vi "Application.vi"(1 "Trial Length (S)":dbl=5.0 min=0.0 step=1.0, 12 "stop (T)":bool=TRUE caption="stop") -> ()   [LabVIEW 2017]
uses:
  <vilib>/addons/_NISVFA/_Shared subVIs/Controls/svc_Window [Dual FFT].ctl
  <vilib>/DAQmx/read.llb/DAQmx Read (Analog 1D DBL NChan 1Samp).vi
  <vilib>/DAQmx/configure/timing.llb/DAQmx Timing (Sample Clock).vi
  <vilib>/DAQmx/create/channels.llb/DAQmx Create Channel (AI-Voltage-Basic).vi
panel:
  in  "Tab Control 5":enum32{"Acquisition", "Results"}(tab)
  out "elapsed time":dbl format="%.2f"
  in  "Lead In":tag="Dev2/ai0"
  in  "Lead Out":tag="Dev2/ai1"
  in  "Trail Out":tag="Dev2/ai3"
  in  "Trail In":tag="Dev2/ai2"
  in  "simulation":bool=TRUE caption="sample clock"
  out "file preview":string
  out "Progress %":dbl(slide) scale=0.0..100.0
  in  "Acquisition Source":enum32{"Device Acquistion", "File Input"}(radio)
  out "Write Path":path
  out "timestamp":string
  in  "file name":string
  out "ai0 Chart":dbl(graph)
  out "ai1 Chart":dbl(graph)
  out "ai2 Chart":dbl(graph)
  out "ai3 Chart":dbl(graph)
  in  "Tab Control":T1(tab)
  out "Raw Signal TA":waveform(dbl)(graph) caption="Waveform Graph"
  out "FFT TA":cluster{"X":dbl, "Y":dbl}[](graph)
  out "dB On 6":bool=TRUE
  out "unit label 9":string
  out "frequency range 8":T2={"low band"=enum."20 Hz", "high band"=enum."20000 Hz"}
  out "octave graph":T3(graph)
  out "total band power [dB] 4":dbl=nan format="%.9f"
  out "RMS [V^2]\nBands [Hz] 5":dbl[][](array[numeric])
  out "unit label":string
  out "frequency range 9":T2={"low band"=enum."20 Hz", "high band"=enum."20000 Hz"}
  out "dB On  2":bool=TRUE
  out "octave graph 2":T3(graph)
  out "total band power [dB EU]":dbl=nan format="%.2f"
  out "SPL [dB]\nBands [Hz]":dbl[][](array[numeric])
  out "SPL [dB] TA":dbl
  out "RMS FFT TA":dbl
  out "Trailing Edge Probe – Mic A":string
  out "Trailing Edge Probe – Mic B":string
  out "Leading Edge Probe – Mic A":string
  out "Leading Edge Probe – Mic B":string
  in  "Tab Control 3":T4(tab) caption="Tab Control"
  out "Raw Signal LA 2":waveform(dbl)(graph) caption="Waveform Graph"
  out "FFT LA":cluster{"X":dbl, "Y":dbl}[](graph)
  out "unit label":string
  out "frequency range RMS 3":T2={"low band"=enum."20 Hz", "high band"=enum."20000 Hz"}
  out "dB On":bool=TRUE
  out "octave graph":T3(graph)
  out "RMS [V^2]\nBands [Hz]":dbl[][](array[numeric])
  out "total band power [dB]":dbl=nan format="%.7f"
  out "unit label":string
  out "dB On 7":bool=TRUE
  out "frequency range":T2={"low band"=enum."20 Hz", "high band"=enum."20000 Hz"}
  out "octave graph 5":T3(graph)
  out "SPL [dB]\nBands [Hz]":dbl[][](array[numeric])
  out "total band power [dB EU]":dbl=nan format="%.2f"
  out "SPL [dB] LA 2":dbl
  out "RMS FFT LA":dbl
  in  "Tab Control 4":T4(tab) caption="Tab Control"
  out "Raw Signal LB":waveform(dbl)(graph) caption="Waveform Graph"
  out "FFT LB":cluster{"X":dbl, "Y":dbl}[](graph)
  out "unit label 10":string
  out "dB On 2":bool=TRUE
  out "frequency range":T2={"low band"=enum."20 Hz", "high band"=enum."20000 Hz"}
  out "octave graph 8":T3(graph)
  out "RMS [V^2]\nBands [Hz]":dbl[][](array[numeric])
  out "total band power [V^2]":dbl=nan format="%.7f"
  out "dB On":bool=TRUE
  out "frequency range":T2={"low band"=enum."20 Hz", "high band"=enum."20000 Hz"}
  out "unit label 11":string
  out "octave graph 7":T3(graph)
  out "SPL [dB]\nBands [Hz] 2":dbl[][](array[numeric])
  out "total band power [dB]":dbl=nan format="%.2f"
  out "SPL [dB] LB":dbl
  out "RMS FFT LB":dbl
  in  "Select Probe:":string(combo)
  out "DATA":string
  out "Single Probe SPL Log Avg:":dbl[][](array[numeric])
  out "Single Probe Coherence [dB EU]":dbl[](array[numeric]) format="%_9g"
  out "Entire-Spectrum Single-Probe SPL [dB]":dbl
  out "Overall SPL Log Avg:":dbl[][](array[numeric])
  out "Entire-Spectrum Overall SPL [dB]:":dbl
  in  "Tab Control 2":T4(tab) caption="Tab Control"
  out "Raw Signal TB":waveform(dbl)(graph) caption="Waveform Graph"
  out "FFT TB":cluster{"X":dbl, "Y":dbl}[](graph)
  out "unit label":string
  out "dB On 5":bool=TRUE
  out "frequency range":T2={"low band"=enum."20 Hz", "high band"=enum."20000 Hz"}
  out "octave graph":T3(graph)
  out "total band power [dB EU]":dbl=nan format="%.7f"
  out "RMS [V^2]\nBands [Hz]":dbl[][](array[numeric])
  out "unit label":string
  out "dB On":bool=TRUE
  out "frequency range":T2={"low band"=enum."20 Hz", "high band"=enum."20000 Hz"}
  out "octave graph":T3(graph)
  out "SPL [dB]\nBands [Hz]":dbl[][](array[numeric])
  out "total band power [dB EU]":dbl=nan format="%.2f"
  out "SPL [dB] TB":dbl
  out "RMS FFT TB":dbl
  out "octave spectrum 4":T5 {"band power" format="%.2f"; "nominal frequencies [Hz]" format="%.2f"}
  # "SPL [dB]"
  # "Band [Hz]"
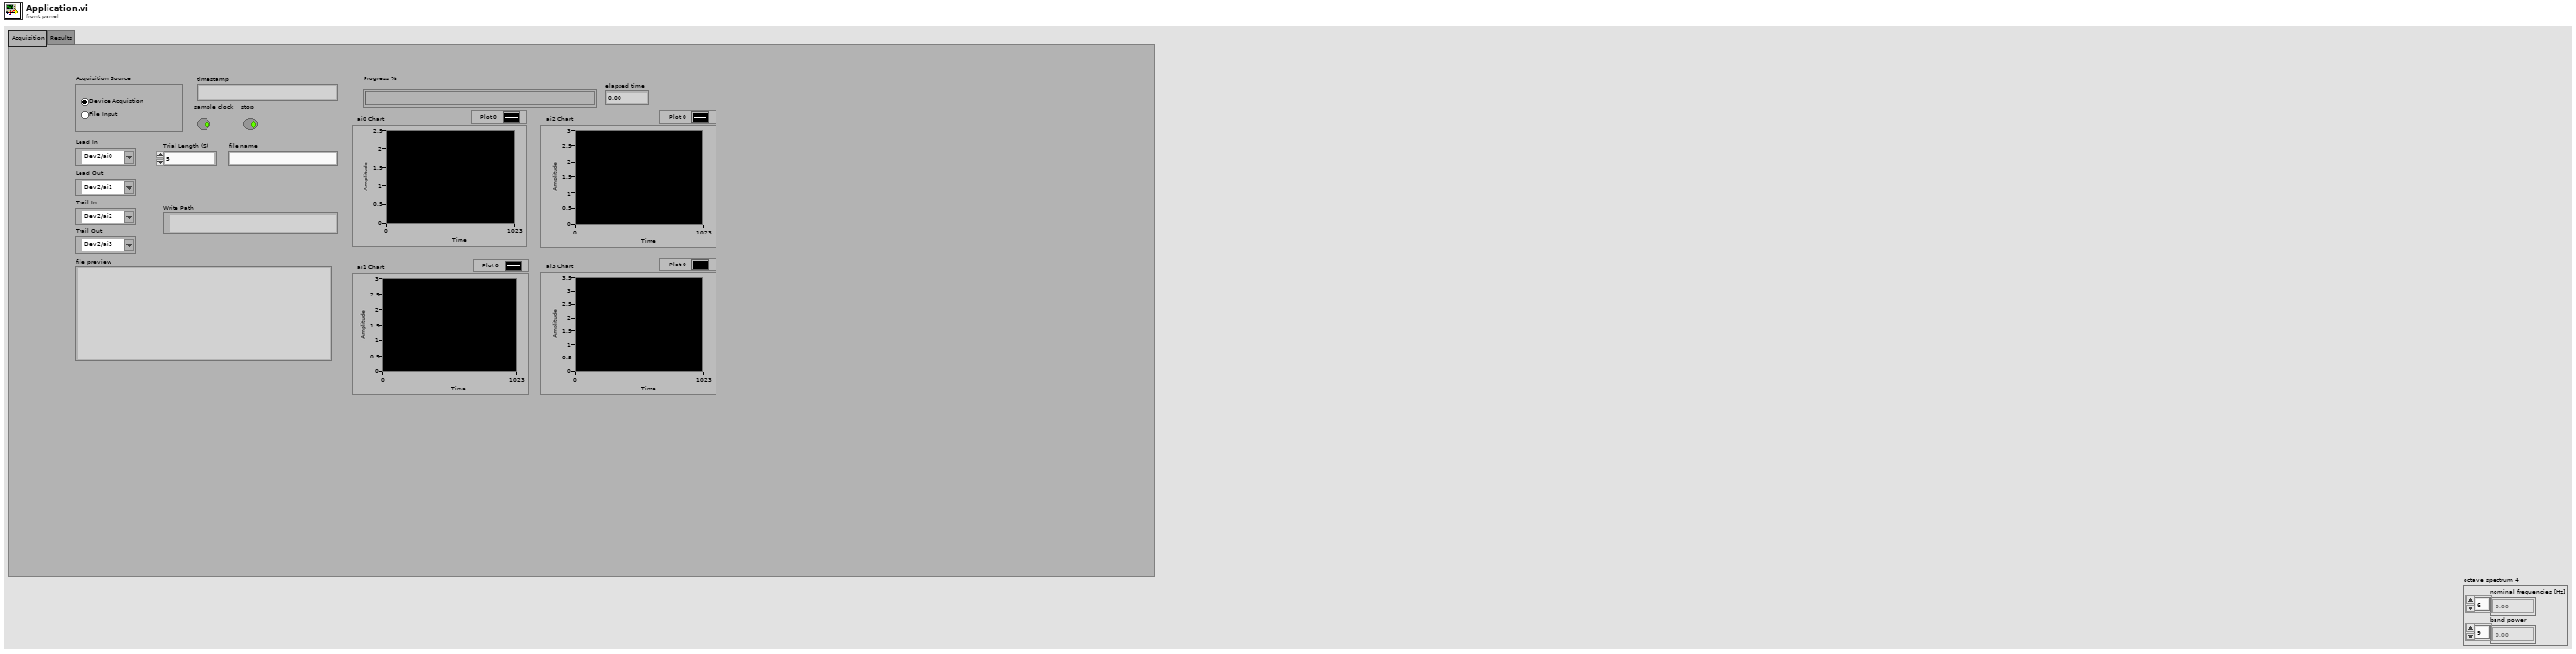
[diagram p1: front panel]
types:
  T1 = enum32{"Raw Signal", "FFT", "FFT Phase", "RMS Graph", "RMS Data", "SPL Graph", "SPL Data", "Full Spectrum Data"}
  T2 = cluster{"low band":enum16{"20 Hz", "25 Hz", "31.5 Hz", "40 Hz", "50 Hz", "63 Hz", "80 Hz", "100 Hz", "125 Hz", "160 Hz", "200 Hz", "250 Hz", "315 Hz", "400 Hz", "500 Hz", "630 Hz", "800 Hz", "1000 Hz", "1250 Hz", "1600 Hz", "2000 Hz", "2500 Hz", "3150 Hz", "4000 Hz", "5000 Hz", "6300 Hz", "8000 Hz", "10000 Hz", "12500 Hz", "16000 Hz", "20000 Hz"}, "high band":enum16{"20 Hz", "25 Hz", "31.5 Hz", "40 Hz", "50 Hz", "63 Hz", "80 Hz", "100 Hz", "125 Hz", "160 Hz", "200 Hz", "250 Hz", "315 Hz", "400 Hz", "500 Hz", "630 Hz", "800 Hz", "1000 Hz", "1250 Hz", "1600 Hz", "2000 Hz", "2500 Hz", "3150 Hz", "4000 Hz", "5000 Hz", "6300 Hz", "8000 Hz", "10000 Hz", "12500 Hz", "16000 Hz", "20000 Hz"}}
  T3 = cluster{"nominal frequencies [Hz]":dbl[], "band power [dB EU]":dbl[]}
  T4 = enum32{"Raw Signal", "FFT", "RMS Graph", "RMS Data", "SPL Graph", "SPL Data", "Full Spectrum Data"}
  T5 = cluster{"nominal frequencies [Hz]":dbl[], "band power":dbl[]}
  T6 = enum16{"Linear", "Exponential", "Equal confidence", "Peak"}
  T7 = typedef "svc_Window [Dual FFT].ctl" = u32
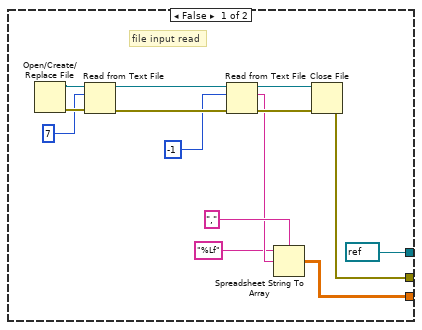
[diagram p2: hidden frame]
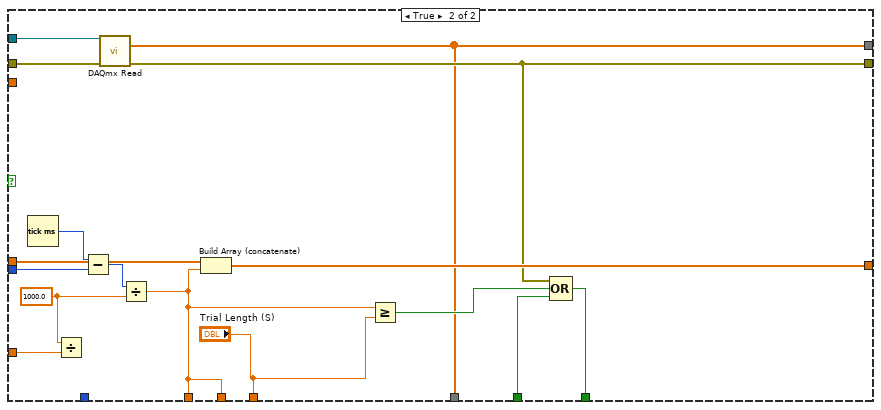
[diagram p4: hidden frame]
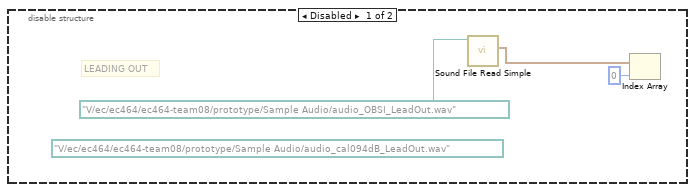
[diagram p6: hidden frame]
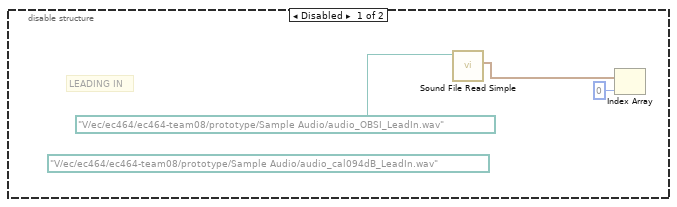
[diagram p7: hidden frame]
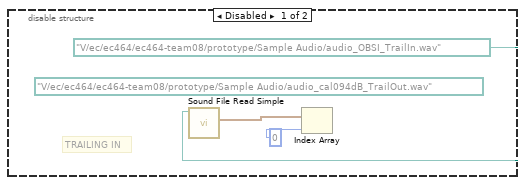
[diagram p9: hidden frame]
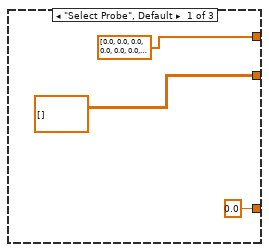
[diagram p10: hidden frame]
diagram:
  n1 = flat-sequence {
    tunnel: [w31] -> w2
    tunnel: [w30] -> w1
    tunnel: [w56] -> w12
    tunnel: [w55] -> w10
    tunnel: [w54] -> w8
    tunnel: [w53] -> w6
    tunnel: [w52] -> w4
    tunnel: w2 -> [w51]
    tunnel: w1 -> [w50]
    tunnel: [w98] -> w14
    tunnel: [w97] -> w13
    tunnel: w12 -> [w97]
    tunnel: [w96] -> w11
    tunnel: w10 -> [w96]
    tunnel: [w95] -> w9
    tunnel: w8 -> [w95]
    tunnel: [w94] -> w7
    tunnel: w6 -> [w94]
    tunnel: [w93] -> w5
    tunnel: w4 -> [w93]
    tunnel: [w92] -> w3
    tunnel: [w118] -> w29
    tunnel: [w117] -> w28
    tunnel: [w113] -> w27
    tunnel: [w116] -> w23
    tunnel: [w115] -> w22
    tunnel: [w114] -> w18
    tunnel: [w111] -> w15
    tunnel: w14 -> [w111]
    tunnel: w13 -> [w110]
    tunnel: w11 -> [w109]
    tunnel: w9 -> [w108]
    tunnel: w7 -> [w107]
    tunnel: w5 -> [w106]
    tunnel: w3 -> [w105]
    tunnel: w29 -> [w188]
    tunnel: [w188] -> w24
    tunnel: [w187] -> w25
    tunnel: w28 -> [w187]
    tunnel: w27 -> [w186]
    tunnel: [w186] -> w26
    tunnel: w23 -> [w185]
    tunnel: w22 -> [w181]
    tunnel: w18 -> [w184]
    tunnel: [w184] -> w17
    tunnel: [w183] -> w16
    tunnel: w15 -> [w183]
    tunnel: [w332] -> w21
    tunnel: [w331] -> w20
    tunnel: [w330] -> w19
    tunnel: w16 -> [w214]
    tunnel: w17 -> [_]
    tunnel: w24 -> [w330]
    tunnel: w25 -> [w331]
    tunnel: w26 -> [w332]
    tunnel: w21 -> [w358]
    tunnel: w20 -> [w359]
    tunnel: w19 -> [w356]
    frame #0 {
      w43 = 0 ("index")
      n2 = call <vilib>:"DAQmx Unflatten Channel String.vi"("names in"="Trail Out") -> ("names out"=w44:string[])  [unwired: 13 in, 1 out]
      n3 = call <vilib>:"DAQmx Unflatten Channel String.vi"("names in"="Trail In") -> ("names out"=w45:string[])  [unwired: 13 in, 1 out]
      n4 = call <vilib>:"DAQmx Unflatten Channel String.vi"("names in"="Lead In") -> ("names out"=w47:string[])  [unwired: 13 in, 1 out]
      n5 = call <vilib>:"DAQmx Unflatten Channel String.vi"("names in"="Lead Out") -> ("names out"=w46:string[])  [unwired: 13 in, 1 out]
      n6 = Index Array(array=w46, index=w43) -> (element=w41:string)
      n7 = Index Array(array=w45, index=w43) -> (element=w40:string)
      n8 = Index Array(array=w47, index=w43) -> (element=w42:string)
      n9 = Index Array(array=w44, index=w43) -> (element=w39:string)
      n10 = call "append channels"("Trail Out"=w39, "Lead In"=w42, "Lead Out"=w41, "Trail In"=w40) -> ("Result"=w31:string, "error out"=w30:errorcluster)  [unwired: 10 in]
      "Trailing Edge Probe – Mic A" <- "Trailing Edge Probe – Mic A"
      "Trailing Edge Probe – Mic B" <- "Trailing Edge Probe – Mic B"
      "Leading Edge Probe – Mic A" <- "Leading Edge Probe – Mic A"
      "Leading Edge Probe – Mic B" <- "Leading Edge Probe – Mic B"
      "DATA" <- "DATA" ("DATA")
    }
    frame #1 {
      w52 = 16384.0 ("y")
      n11 = Equal To 0?(x="Acquisition Source") -> (x = 0?=w56:bool)
      n12 = case shown="True" w56 {
        tunnel: [refnum<k21> refnum ("task out") w81] -> w55
        tunnel: [w62 w80] -> w54
        tunnel: w52 -> [_ w76]
        tunnel: [w58 dbl[][] []] -> w53
        tunnel: w51 -> [_ w72]
        tunnel: w50 -> [_ w73]
        frame False {
          # "file input read"
          n13 = Open/Create/Replace File() -> (refnum out=w70:refnum<file>, error out=w69:errorcluster)  [unwired: 6 in, 1 out]
          n14 = Read from Text File(file (use dialog)=w70, count=7, error in=w69) -> (refnum out=w67:refnum<file>, error out=w64:errorcluster)  [unwired: 1 in, 2 out]
          n15 = Read from Text File(file (use dialog)=w67, count=-1, error in=w64) -> (refnum out=w66:refnum<file>, text=w60:string, error out=w65:errorcluster)  [unwired: 1 in, 1 out]
          n16 = Spreadsheet String To Array(delimiter (Tab)=",", format string="%Lf", spreadsheet string=w60) -> (array=w58:dbl[][])  [unwired: 1 in]
          n17 = Close File(refnum=w66, error in=w65) -> (error out=w62:errorcluster)  [unwired: 1 out]
        }
        frame True {
          w79 = 10348 items=["Volts"=10348, "From Custom Scale"=10065] ("units")
          n18 = call-poly <vilib>:"DAQmx Create Virtual Channel.vi"("physical channels"=w72, "units"=w79, "error in"=w73) -> ("task out"=w78:refnum<k21>, "error out"=w77:errorcluster)  [unwired: 11 in]
          n19 = case shown="True" "simulation" {
            tunnel: [w83 w91] -> w81
            tunnel: [w82 w90] -> w80
            tunnel: w78 -> [w83 w89]
            tunnel: w77 -> [w82 w88]
            tunnel: w76 -> [_ w85]
            frame False {
            }
            frame True {
              w87 = 10178 items=["Finite Samples"=10178, "Continuous Samples"=10123, "Hardware Timed Single Point"=12522] ("sample mode")
              n20 = local read "Trial Length (S)"() -> (w86:dbl)
              n21 = Multiply(x=w86, y=w85) -> (x*y=w84:dbl)
              n22 = call-poly <vilib>:"DAQmx Timing.vi"("task/channels in"=w89, "sample mode"=w87, "samples per channel"=w84, "rate"=w85, "error in"=w88) -> ("task out"=w91:refnum<k21>, "error out"=w90:errorcluster)  [unwired: 9 in]
            }
          }
        }
      }
    }
    frame #2 {
      # "Get the timestamp"
      n23 = Get Date/Time In Seconds() -> (seconds since 1Jan1904=w98:timestamp)
      n24 = Tick Count (ms)() -> (millisecond timer value=w92:u32)
      n25 = Get Date/Time String(date format (0)=enum16{"short", "long", "abbreviated"}."long", seconds (now)=w98, want seconds? (F)=TRUE) -> (date string=w102:string, time string=w104:string)
      n26 = call <vilib>:"Space Constant.vi"() -> ("String"=w103:string)
      n27 = Concatenate Strings(w102, w103, w104) -> (→"timestamp":string)
    }
    frame #3 {
      n28 = while {
        shift-right: [w143] -> w117
        shift-left: dbl[] [] -> [w146]
        tunnel: [w137] -> w118 mode=indexing
        tunnel: [w137] -> w114
        tunnel: [w142] -> w115
        tunnel: [w130] -> w113 mode=indexing
        tunnel: w110 -> [w124]
        tunnel: w109 -> [w123]
        tunnel: w108 -> [w122]
        tunnel: w107 -> [w121]
        tunnel: w106 -> [w120]
        tunnel: w105 -> [w119]
        i -> [w137]
        stop <- w144 stop-if-true
        # "TO"
        # "TI"
        # "LO"
        # "LI"
        n29 = case shown="False" w124 {
          tunnel: w146 -> [_ w179]
          tunnel: w119 -> [w153 w169]
          tunnel: "stop (T)" -> [w163 w178]
          tunnel: [w162 w177] -> w144
          tunnel: [w152 w176] -> w143
          tunnel: w123 -> [_ w175]
          tunnel: w122 -> [w164 w174]
          tunnel: [w151 w171] -> w130
          tunnel: [w164 w173] -> w142
          tunnel: w120 -> [_ w172]
          tunnel: [w155 w165] -> w136
          tunnel: [w154 "Trial Length (S)"] -> w140
          tunnel: w121 -> [w160 _]
          tunnel: w137 -> [w155 _]
          tunnel: [w147 w165] -> w135
          tunnel: [w151 w171] -> w129
          frame False {
            # "file input parse"
            n30 = Tick Count (ms)() -> (millisecond timer value=w150:u32)
            n31 = Subtract(x=w150, y=w153) -> (x-y=w149:u32)
            n32 = Divide(x=w149, y=1000.0 ("x")) -> (x/y=w147:dbl)
            n33 = Index Array(array=w160, index (row)=w155) -> (element=w157:dbl[])  [unwired: 1 in]
            n34 = Index Array(array=w160, index (col)=1 ("disabled index (col)")) -> (element=w152:dbl[])  [unwired: 1 in]
            n35 = Array Subset(array=w157, index=2, length=4) -> (w151:dbl[])
            n36 = Array Size(array=w152) -> (size(s)=w154:i32)
            n37 = Greater Or Equal?(x=w155, y=w154) -> (x >= y?=w156:bool)
            n38 = Compound Arithmetic op=OR(w156, w163) -> (w162:bool)
          }
          frame True {
            w167 = 1000.0 ("x")
            n39 = Tick Count (ms)() -> (millisecond timer value=w168:u32)
            n40 = Divide(x=w167, y=w172) -> ()  [unwired: 1 out]
            n41 = Subtract(x=w168, y=w169) -> (x-y=w166:u32)
            n42 = call-poly <vilib>:"DAQmx Read.vi"("task/channels in"=w175, "error in"=w174) -> ("data"=w171:dbl[], "error out"=w173:errorcluster)  [unwired: 11 in, 1 out]
            n43 = Divide(x=w166, y=w167) -> (x/y=w165:dbl)
            n44 = Build Array (concatenate)(w179, w165) -> (w176:dbl[])
            n45 = Greater Or Equal?(x=w165, y="Trial Length (S)") -> (x >= y?=w180:bool)
            n46 = Compound Arithmetic op=OR(w173, w180, w178) -> (w177:bool)
          }
        }
        "elapsed time" <- w135
        n47 = Divide(x=w136, y=w140) -> (x/y=w139:dbl)
        n48 = Multiply(x=w139, y=100.0) -> (x*y=→"Progress %":dbl)
        n49 = Index Array(array=w129, index=2 ("disabled index (col)")) -> (element=→"ai2 Chart":dbl)
        n50 = Index Array(array=w129, index=3 ("disabled index (col)")) -> (element=→"ai3 Chart":dbl)
        n51 = Index Array(array=w129, index=0 ("disabled index (col)")) -> (element=→"ai0 Chart":dbl)
        n52 = Index Array(array=w129, index=1 ("disabled index (col)")) -> (element=→"ai1 Chart":dbl)
      }
      n53 = Equal To 0?(x=w114) -> (x = 0?=w116:bool)
    }
    frame #4 {
      n54 = Compound Arithmetic op=OR(w181, w185) -> (w182:bool)
      n55 = case shown="True" w182 {
        selector: w182 -> [w194 _]
        tunnel: w181 -> [w193 _]
        frame True {
          n56 = And(x=w194, y=w193) -> (x .and. y?=w196:bool)
          n57 = flat-sequence {
            tunnel: [w200] -> w197
            tunnel: w193 -> [w199]
            tunnel: w189 -> [w198]
            tunnel: w197 -> [w202]
            frame #0 {
              n58 = call "Display Message to User2"("error in (no error)"=w199, "Message"=w198) -> ("stop program"=w200:bool)  [unwired: 8 in, 1 out]
            }
            frame #1 {
              n59 = Or(x=TRUE, y=w202) -> (x .or. y?=w203:bool)
              n60 = Stop(stop? (T)=w203) -> ()
            }
          }
          n61 = call <vilib>:"Simple Error Handler.vi"() -> ("message"=w191:string)  [unwired: 5 in, 4 out]
          n62 = Select(t=w191, s=w196, f="Application Stopped, No Error.") -> (s? t:f=w190:string)
          n63 = Concatenate Strings("Application Error: ", w190) -> (w189:string)
        }
        frame False {
        }
      }
    }
    frame #5 {
      w205 = T7 1 items=["None"=0, "Hanning"=1, "Hamming"=2, "Blackman-Harris"=3, "Exact Blackman"=4, "Blackman"=5, "Flat Top"=6, "4 Term B-Harris "=7, "7 Term B-Harris"=8, "Low Sidelobe"=9, "Force - Exponential"=10, "Force"=64, "Exponential"=65, "Blackman Nuttall"=11, "Triangle"=30, "Bartlett-Hanning"=31, "Bohman"=32, "Parzen"=33, "Welch"=34, "Kaiser"=60, "Dolph-Chebyshev"=61, "Gaussian"=62] ("window")
      w207 = T7 1 items=["None"=0, "Hanning"=1, "Hamming"=2, "Blackman-Harris"=3, "Exact Blackman"=4, "Blackman"=5, "Flat Top"=6, "4 Term B-Harris "=7, "7 Term B-Harris"=8, "Low Sidelobe"=9, "Force - Exponential"=10, "Force"=64, "Exponential"=65, "Blackman Nuttall"=11, "Triangle"=30, "Bartlett-Hanning"=31, "Bohman"=32, "Parzen"=33, "Welch"=34, "Kaiser"=60, "Dolph-Chebyshev"=61, "Gaussian"=62] ("window")
      # "dt"
      # "t0"
      # "SPL"
      # "RMS"
      # "LEADING"
      # "OVERALL SPL LOG AVG"
      # "ENTIRE SPECTRUM SINGLE PROBE SPL LOG SUM"
      # "TRAILING"
      # "RMS"
      # "SPL"
      # "ACROSS PROBE AVERAGED SPL"
      # "RMS"
      # "SPL"
      # "ACROSS PROBE AVERAGED SPL"
      # "RMS"
      # "SPL"
      # "TO"
      # "TI"
      # "LO"
      # "LI"
      n64 = Reciprocal(x=16384.0 ("y")) -> (1/x=w211:dbl)
      n65 = disable-structure shown="Enabled" {
        frame Disabled {
          (unwired) path "V:/ec/ec464/ec464-team08/prototype/Sample Audio/audio_cal094dB_TrailOut.wav" ("path")
          # "TRAILING IN"
          n66 = call <vilib>:"Sound File Read Simple.vi"("path"=path "V:/ec/ec464/ec464-team08/prototype/Sample Audio/audio_OBSI_TrailIn.wav") -> ("data"=w342:waveform(dbl)[])  [unwired: 7 in, 3 out]
          n67 = Index Array(array=w342, index=0) -> ()  [unwired: 1 out]
        }
        frame Enabled {
        }
      }
      n68 = Index Array(array=w332, index (col)=0 ("disabled index (col)")) -> (element=w213:dbl[])  [unwired: 1 in]
      n69 = Index Array(array=w332, index (col)=2 ("disabled index (col)")) -> (element=w212:dbl[])  [unwired: 1 in]
      n70 = Index Array(array=w332, index (col)=3 ("disabled index (col)")) -> (element=w209:dbl[])  [unwired: 1 in]
      n71 = Index Array(array=w332, index (col)=1 ("disabled index (col)")) -> (element=w218:dbl[])  [unwired: 1 in]
      n72 = Bundle By Name("t0"=w214, "dt"=w211, "Y"=w213) -> (w215:waveform(dbl))  [unwired: 1 in]
      "Raw Signal LA 2" <- w215
      n73 = Bundle By Name("t0"=w214, "dt"=w211, "Y"=w218) -> (w217:waveform(dbl))  [unwired: 1 in]
      "Raw Signal LB" <- w217
      n74 = Bundle By Name("t0"=w214, "dt"=w211, "Y"=w212) -> (w208:waveform(dbl))  [unwired: 1 in]
      "Raw Signal TA" <- w208
      n75 = Bundle By Name("t0"=w214, "dt"=w211, "Y"=w209) -> (w210:waveform(dbl))  [unwired: 1 in]
      "Raw Signal TB" <- w210
      n76 = call "EntireSpectrumProcess.vi"("data"=w208) -> ("RMS"=→"RMS FFT TA":dynamicdata, "Dynamic Data"=→"SPL [dB] TA":dynamicdata, "Array"=→"FFT TA":cluster{dbl, dbl}[])  [unwired: 8 in]
      n77 = call "OctaveBandsProcess.vi"("averaging type"=T6."Linear", "data"=w208, "dB On (T)"=FALSE) -> ("nominal frequencies [Hz]"=w309:dbl[], "frequency range"=→"frequency range 8":T2, "band power"=w289:dbl[], "octave spectrum"=→"octave graph":T5, "dB On"=→"dB On 6":bool, "unit label"=w287:string, "total band power"=→"total band power [dB] 4":dbl)  [unwired: 5 in, 1 out]
      "unit label 9" <- w287
      n78 = call "OctaveBandsProcess.vi"("averaging type"=T6."Linear", "data"=w208, "dB On (T)"=TRUE) -> ("nominal frequencies [Hz]"=w298:dbl[], "frequency range"=→"frequency range 9":T2, "band power"=w291:dbl[], "octave spectrum"=→"octave graph 2":T5, "dB On"=→"dB On  2":bool, "unit label"=w281:string, "total band power"=→"total band power [dB EU]":dbl)  [unwired: 5 in, 1 out]
      "unit label" <- w281
      n79 = property on="octave graph 2" class="XYGraph (strict)"("Y Scale.Name Label.Text"=w281) -> ()  [unwired: 2 in, 2 out]
      n80 = property on="octave graph" class="XYGraph (strict)"("Y Scale.Name Label.Text"=w287) -> ()  [unwired: 2 in, 2 out]
      n81 = disable-structure shown="Disabled" {
        frame Disabled {
          (unwired) path "V:/ec/ec464/ec464-team08/prototype/Sample Audio/audio_cal094dB_TrailOut.wav" ("path")
          # "TRAILING OUT"
          n82 = call <vilib>:"Sound File Read Simple.vi"("path"=path "V:/ec/ec464/ec464-team08/prototype/Sample Audio/audio_OBSI_TrailOut.wav") -> ("data"=w339:waveform(dbl)[])  [unwired: 7 in, 3 out]
          n83 = Index Array(array=w339, index=0) -> ()  [unwired: 1 out]
        }
        frame Enabled {
        }
      }
      n84 = Build Array(w291, w298) -> (→"SPL [dB]\nBands [Hz]":dbl[][])
      n85 = Build Array(w289, w309) -> (→"RMS [V^2]\nBands [Hz] 5":dbl[][])
      n86 = call "OctaveBandsProcess.vi"("averaging type"=T6."Linear", "data"=w210, "dB On (T)"=FALSE) -> ("nominal frequencies [Hz]"=w306:dbl[], "frequency range"=→"frequency range":T2, "band power"=w290:dbl[], "octave spectrum"=→"octave graph":T5, "dB On"=→"dB On 5":bool, "unit label"=w272:string, "total band power"=→"total band power [dB EU]":dbl)  [unwired: 5 in, 1 out]
      "unit label" <- w272
      n87 = call <vilib>:"SVFA Coherent Output Power.vi"("scaled signal X [EUx]"=w289, "scaled signal Y [EUy]"=w290, "window"=w205) -> ("coherent output power [dB EUy]"=w204:cluster{"f0":dbl, "df":dbl, "magnitude":dbl[]})  [unwired: 10 in, 6 out]
      n88 = Unbundle(w204) -> ("magnitude"=w221:dbl[])  [unwired: 2 out]
      n89 = call "OctaveBandsProcess.vi"("averaging type"=T6."Linear", "data"=w210, "dB On (T)"=TRUE) -> ("nominal frequencies [Hz]"=w307:dbl[], "frequency range"=→"frequency range":T2, "band power"=w308:dbl[], "octave spectrum"=→"octave graph":T5, "dB On"=→"dB On":bool, "unit label"=w266:string, "total band power"=→"total band power [dB EU]":dbl)  [unwired: 5 in, 1 out]
      "unit label" <- w266
      n90 = call "LogAverage.vi"("band power 2"=w291, "band power"=w308) -> ("Array"=w296:dbl[])  [unwired: 9 in]
      n91 = Build Array(w296, w298) -> (w297:dbl[][])
      n92 = call "EntireSpectrumProcess.vi"("data"=w210) -> ("RMS"=→"RMS FFT TB":dynamicdata, "Dynamic Data"=→"SPL [dB] TB":dynamicdata, "Array"=→"FFT TB":cluster{dbl, dbl}[])  [unwired: 8 in]
      n93 = property on="octave graph" class="XYGraph (strict)"("Y Scale.Name Label.Text"=w266) -> ()  [unwired: 2 in, 2 out]
      n94 = property on="octave graph" class="XYGraph (strict)"("Y Scale.Name Label.Text"=w272) -> ()  [unwired: 2 in, 2 out]
      n95 = Build Array(w290, w306) -> (→"RMS [V^2]\nBands [Hz]":dbl[][])
      n96 = disable-structure shown="Enabled" {
        frame Disabled {
          (unwired) path "V:/ec/ec464/ec464-team08/prototype/Sample Audio/audio_cal094dB_LeadIn.wav" ("path")
          # "LEADING IN"
          n97 = call <vilib>:"Sound File Read Simple.vi"("path"=path "V:/ec/ec464/ec464-team08/prototype/Sample Audio/audio_OBSI_LeadIn.wav") -> ("data"=w338:waveform(dbl)[])  [unwired: 7 in, 3 out]
          n98 = Index Array(array=w338, index=0) -> ()  [unwired: 1 out]
        }
        frame Enabled {
        }
      }
      n99 = Build Array(w308, w307) -> (→"SPL [dB]\nBands [Hz]":dbl[][])
      n100 = call "LogSum.vi"("Array"=w296) -> ("Numeric"=w295:dbl)  [unwired: 10 in]
      n101 = call "EntireSpectrumProcess.vi"("data"=w215) -> ("RMS"=→"RMS FFT LA":dynamicdata, "Dynamic Data"=→"SPL [dB] LA 2":dynamicdata, "Array"=→"FFT LA":cluster{dbl, dbl}[])  [unwired: 8 in]
      n102 = call "OctaveBandsProcess.vi"("averaging type"=T6."Linear" ("averaging type 4"), "data"=w215, "dB On (T)"=FALSE) -> ("nominal frequencies [Hz]"=w303:dbl[], "frequency range"=→"frequency range RMS 3":T2, "band power"=w223:dbl[], "octave spectrum"=→"octave graph":T5, "dB On"=→"dB On":bool, "unit label"=w257:string, "total band power"=→"total band power [dB]":dbl)  [unwired: 5 in, 1 out]
      "unit label" <- w257
      n103 = call "OctaveBandsProcess.vi"("averaging type"=T6."Linear", "data"=w215, "dB On (T)"=TRUE) -> ("nominal frequencies [Hz]"=w304:dbl[], "frequency range"=→"frequency range":T2, "band power"=w305:dbl[], "octave spectrum"=→"octave graph 5":T5, "dB On"=→"dB On 7":bool, "unit label"=w251:string, "total band power"=→"total band power [dB EU]":dbl)  [unwired: 5 in, 1 out]
      "unit label" <- w251
      n104 = disable-structure shown="Enabled" {
        frame Disabled {
          (unwired) path "V:/ec/ec464/ec464-team08/prototype/Sample Audio/audio_cal094dB_LeadOut.wav" ("path")
          # "LEADING OUT"
          n105 = call <vilib>:"Sound File Read Simple.vi"("path"=path "V:/ec/ec464/ec464-team08/prototype/Sample Audio/audio_OBSI_LeadOut.wav") -> ("data"=w335:waveform(dbl)[])  [unwired: 7 in, 3 out]
          n106 = Index Array(array=w335, index=0) -> ()  [unwired: 1 out]
        }
        frame Enabled {
        }
      }
      n107 = property on="octave graph 5" class="XYGraph (strict)"("Y Scale.Name Label.Text"=w251) -> ()  [unwired: 2 in, 2 out]
      n108 = property on="octave graph" class="XYGraph (strict)"("Y Scale.Name Label.Text"=w257) -> ()  [unwired: 2 in, 2 out]
      n109 = Build Array(w223, w303) -> (→"RMS [V^2]\nBands [Hz]":dbl[][])
      n110 = Build Array(w305, w304) -> (→"SPL [dB]\nBands [Hz]":dbl[][])
      n111 = call "EntireSpectrumProcess.vi"("data"=w217) -> ("RMS"=→"RMS FFT LB":dynamicdata, "Dynamic Data"=→"SPL [dB] LB":dynamicdata, "Array"=→"FFT LB":cluster{dbl, dbl}[])  [unwired: 8 in]
      n112 = call "OctaveBandsProcess.vi"("averaging type"=T6."Linear" ("averaging type 6"), "data"=w217, "dB On (T)"=FALSE) -> ("nominal frequencies [Hz]"=w302:dbl[], "frequency range"=→"frequency range":T2, "band power"=w222:dbl[], "octave spectrum"=→"octave graph 8":T5, "dB On"=→"dB On 2":bool, "unit label"=w242:string, "total band power"=→"total band power [V^2]":dbl)  [unwired: 5 in, 1 out]
      "unit label 10" <- w242
      n113 = call <vilib>:"SVFA Coherent Output Power.vi"("scaled signal X [EUx]"=w223, "scaled signal Y [EUy]"=w222, "window"=w207) -> ("coherent output power [dB EUy]"=w206:cluster{"f0":dbl, "df":dbl, "magnitude":dbl[]})  [unwired: 10 in, 6 out]
      n114 = Unbundle(w206) -> ("magnitude"=w220:dbl[])  [unwired: 2 out]
      n115 = call "OctaveBandsProcess.vi"("averaging type"=T6."Linear", "data"=w217, "dB On (T)"=TRUE) -> ("nominal frequencies [Hz]"=w300:dbl[], "frequency range"=→"frequency range":T2, "band power"=w301:dbl[], "octave spectrum"=→"octave graph 7" →"octave spectrum 4":T5, "dB On"=→"dB On":bool, "unit label"=w236:string, "total band power"=→"total band power [dB]":dbl)  [unwired: 5 in, 1 out]
      "unit label 11" <- w236
      n116 = call "LogAverage.vi"("band power 2"=w305, "band power"=w301) -> ("Array"=w293:dbl[])  [unwired: 9 in]
      n117 = call "LogSum.vi"("Array"=w293) -> ("Numeric"=w294:dbl)  [unwired: 10 in]
      n118 = call "LogAverage.vi"("band power 2"=w293, "band power"=w296) -> ("Array"=w292:dbl[])  [unwired: 9 in]
      n119 = Build Array(w292, w298) -> (→"Overall SPL Log Avg:":dbl[][])
      n120 = call "LogSum.vi"("Array"=w292) -> ("Numeric"=→"Entire-Spectrum Overall SPL [dB]:":dbl)  [unwired: 10 in]
      n121 = Build Array(w293, w304) -> (w299:dbl[][])
      n122 = case shown="\"Trailing Edge Probe\"" "Select Probe:" {
        tunnel: w297 -> [_ w350 _]
        tunnel: [dbl[][] [] w350 w353] -> w227
        tunnel: w299 -> [_ _ w353]
        tunnel: w295 -> [_ w349 _]
        tunnel: [0.0 ("Numeric") w349 w352] -> w226
        tunnel: w294 -> [_ _ w352]
        tunnel: w221 -> [_ w348 _]
        tunnel: w220 -> [_ _ w351]
        tunnel: [dbl[] [0.0, 0.0, 0.0, 0.0, 0.0, 0.0, 0.0] ("Single Probe Coherence [dB EU]") w348 w351] -> w219
        frame "Select Probe", Default {
        }
        frame "Trailing Edge Probe" {
        }
        frame "Leading Edge Probe" {
        }
      }
      "Single Probe SPL Log Avg:" <- w227
      "Entire-Spectrum Single-Probe SPL [dB]" <- w226
      "Single Probe Coherence [dB EU]" <- w219
      n123 = property on="octave graph 7" class="XYGraph (strict)"("Y Scale.Name Label.Text"=w236) -> ()  [unwired: 2 in, 2 out]
      n124 = property on="octave graph 8" class="XYGraph (strict)"("Y Scale.Name Label.Text"=w242) -> ()  [unwired: 2 in, 2 out]
      n125 = Build Array(w222, w302) -> (→"RMS [V^2]\nBands [Hz]":dbl[][])
      n126 = Build Array(w301, w300) -> (→"SPL [dB]\nBands [Hz] 2":dbl[][])
    }
    frame #6 {
      n127 = Transpose 2D Array(2D array=w358) -> (transposed array=w357:dbl[][])
      n128 = Build Array (concatenate)(w359, w357) -> (w355:dbl[][])
      n129 = Two Button Dialog(message="Save to File?", 1:"No" ("F button name (\"Cancel\")"), 2:"Yes" ("T button name (\"OK\")")) -> (T button?=w363:bool)
      n130 = Transpose 2D Array(2D array=w355) -> (transposed array=w354:dbl[][])
      n131 = case shown="True" w363 {
        tunnel: w354 -> [_ w388]
        tunnel: w356 -> [_ w387]
        frame False {
        }
        frame True {
          # "writing raw file data"
          # "Writeback\n\nFile Format for CSV:\n\nFilename\nTimestamp\nSystem Info (OS, build, etc)\nTime duration\nNumber of entries"
          n132 = for {
            tunnel: w388 -> [w393] mode=indexing
            tunnel: w387 -> [w392] mode=indexing
            tunnel: [w391] -> w375 mode=indexing
            n133 = Number To Decimal String(number=w392) -> (decimal integer string=w395:string)  [unwired: 1 in]
            n134 = Array To Spreadsheet String(delimiter (Tab)=",", array=w393, 3:"%f" ("format string")) -> (spreadsheet string=w390:string)
            n135 = call <vilib>:"Trim Whitespace.vi"("string"=w390) -> ("trimmed string"=w389:string)  [unwired: 1 in]
            n136 = Concatenate Strings(w395, "," ("delimiter (Tab)"), w389) -> (w391:string)
          }
          n137 = Equal?(x="file name", y="") -> (x = y?=w381:bool)
          n138 = Select(t="unnamed_raw_acquisition", s=w381, f="file name") -> (s? t:f=w378:string)
          n139 = Concatenate Strings(w378, ".csv" ("string")) -> (w377:string)
          n140 = local read "timestamp"() -> (w372:string)
          n141 = Array To Spreadsheet String(delimiter (Tab)="\r\n", array=w375, 3:"%s" ("format string")) -> (spreadsheet string=w366:string)
          n142 = Concatenate Strings("File name: " ("string"), w377) -> (w373:string)
          n143 = CPU Information() -> (4:w371:i32, 5:w370:i32, 6:w369:i32, 7:w368:i32)
          n144 = call "create string file"("Beginning Text"="", "packages"=w370, "logical processors"=w368, "file name"=w373, "timestamp"=w372, "processors"=w371, "core per package"=w369, "data"=w366) -> ("Result"=w367:string)  [unwired: 6 in, 1 out]
          "file preview" <- w367
          n145 = call "WriteToFile.vi"("Write to file"=TRUE, "sub folder"="runs", "Output File"=w377, "contents"=w367) -> ("path"=→"Write Path":path)  [unwired: 6 in, 1 out]
        }
      }
    }
  }
